vi "Process.vi"(8 "error in":errorcluster, 11 "Plugin in":refnum<class "Sequencer with Output Values.lvclass">) -> (0 "error out":errorcluster, 3 "Plugin out":refnum<class "Sequencer with Output Values.lvclass">)   [LabVIEW 2024, in "Sequencer with Output Values.lvlib" / "Sequencer with Output Values.lvclass"]
uses:
  Sequencer with Output Values.lvclass
  C:/Program Files/National Instruments/LabVIEW 2024/vi.lib/FlexLogger/SDK/PluginSDK.lvlibp/PEFClasses/SDK/Plugin/Plugin.lvclass
  Sequencer with Output Values.lvclass/Sequencer with Output Values.ctl
  <vilib>/FlexLogger/SDK/PluginSDK.lvlibp/PEFClasses/SDK/Plugin/DataHelpers/Write 1D DBL (NChan 1Sample).vi
  <vilib>/FlexLogger/SDK/PluginSDK.lvlibp/PEFClasses/SDK/Plugin/DataHelpers/Write 1D Bool (NChan 1 Sample).vi
  <vilib>/FlexLogger/SDK/PluginSDK.lvlibp/PEFClasses/SDK/Plugin/Plugin.lvclass
  C:/Program Files/National Instruments/LabVIEW 2024/vi.lib/FlexLogger/SDK/PluginSDK.lvlibp/PEFClasses/SDK/Processing Element/Processing Element.lvclass
  C:/dev/niflexlogger-plugins/plugins/Sequencer with Output Values/source/Sequencer with Output Values/Sequencer with Output Values.lvclass
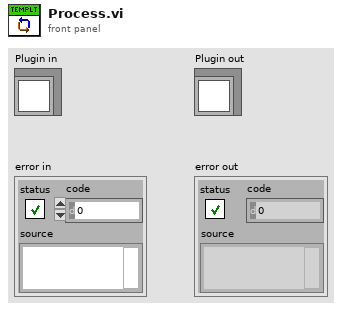
[diagram p1: front panel]
types:
  T1 = typedef "Sequencer with Output Values.lvlib/Sequencer with Output Values.lvclass/Params.ctl" = cluster{"Step Values":T2[], "Only Execute When Test Running":bool, "Current Sequence ID":u32, "Total Iterations":u32, "Last Timestamp":timestamp, "Number of Sequence Steps":i32, "Number of Analog Channels":i32, "Number of Digital Channels":i32, "Delay Before Starting Sequence":dbl}
  T2 = typedef "Step Settings.ctl" = cluster{"Duration":dbl, "Mode":string, "Delay Between Values":dbl, "Analog Values":string[], "Digital Values":string[]}
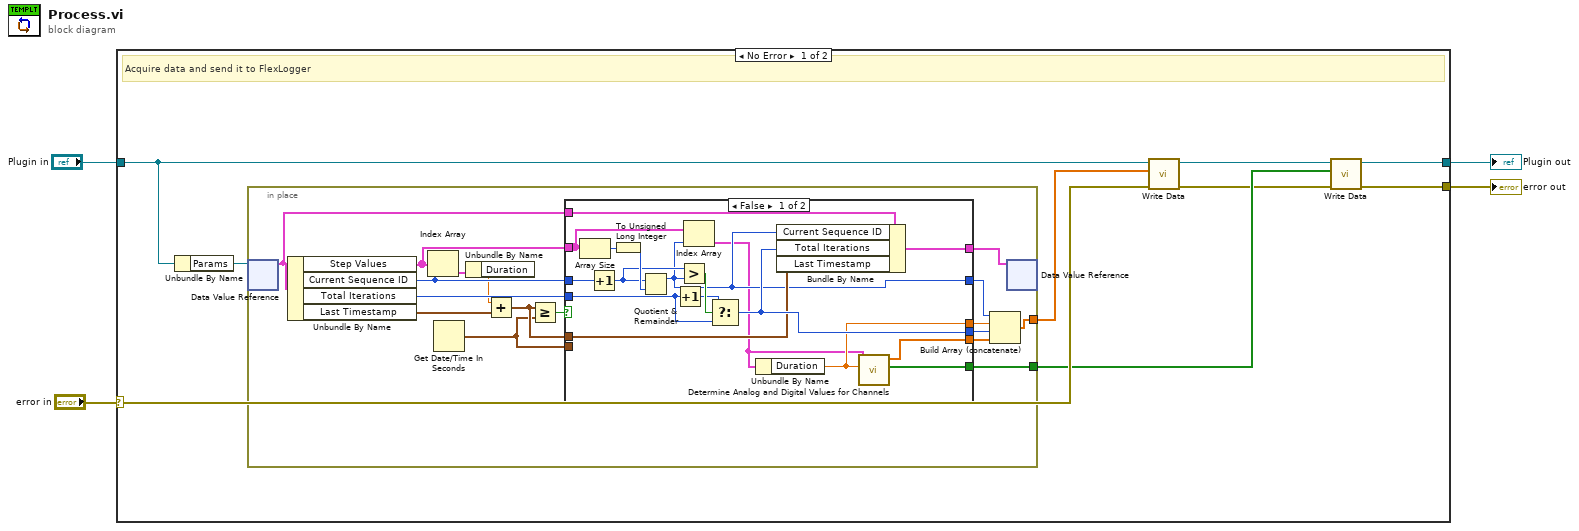
[diagram p0: block diagram]
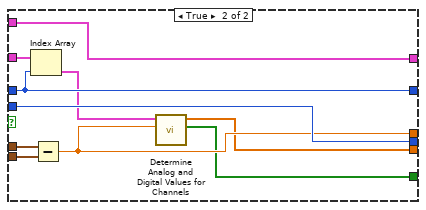
[diagram p2: hidden frame]
diagram:
  n1 = case shown="No Error" "error in" {
    selector: "error in" -> [w12 w58]
    tunnel: [w6 w59] -> w4
    tunnel: "Plugin in" -> [w13 w59]
    tunnel: [w5 w58] -> w1
    frame No Error {
      # "Acquire data and send it to FlexLogger"
      n2 = Unbundle By Name(w13) -> ("Params"=w11:refnum<data-value>)
      n3 = in-place {
        in-place-border: [w27] -> w10
        in-place-border: [w14] -> w8
        n4 = in-place-dvr #1(w11) -> (w30:T1)  [unwired: 1 out]
        n5 = Unbundle By Name(w30) -> ("Step Values"=w29:T2[], "Current Sequence ID"=w25:u32, "Total Iterations"=w28:u32, "Last Timestamp"=w23:timestamp)
        n6 = Index Array(array=w29, index=w25) -> (element=w21:T2)
        n7 = Get Date/Time In Seconds() -> (seconds since 1Jan1904=w17:timestamp)
        n8 = Unbundle By Name(w21) -> ("Duration"=w20:dbl)
        n9 = Add(x=w20, y=w23) -> (x+y=w18:timestamp)
        n10 = Greater Or Equal?(x=w18, y=w17) -> (x >= y?=w24:bool)
        n11 = case shown="False" w24 {
          tunnel: w30 -> [w42 w56]
          tunnel: w25 -> [w46 w52]
          tunnel: w29 -> [w36 w53]
          tunnel: w28 -> [w44 w57]
          tunnel: [w35 w52] -> w22
          tunnel: [w40 w57] -> w19
          tunnel: [w41 w56] -> w26
          tunnel: w18 -> [w37 w55]
          tunnel: w17 -> [_ w54]
          tunnel: [w32 w50] -> w16
          tunnel: [w34 w49] -> w15
          tunnel: [w33 w48] -> w14
          frame False {
            n12 = Array Size(array=w36) -> (size(s)=w47:i32)
            n13 = Increment(x=w46) -> (x+1=w38:u32)
            n14 = To Unsigned Long Integer(number=w47) -> (unsigned 32bit integer=w39:u32)
            n15 = Quotient & Remainder(x=w38, y=w39) -> (x-y*floor(x/y)=w35:u32)  [unwired: 1 out]
            n16 = Increment(x=w44) -> (x+1=w43:u32)
            n17 = Greater?(x=w38, y=w35) -> (0:w45:bool)
            n18 = Index Array(array=w36, index=w35) -> (element=w31:T2)
            n19 = Select(t=w43, s=w45, f=w44) -> (s? t:f=w40:u32)
            n20 = Unbundle By Name(w31) -> ("Duration"=w32:dbl)
            n21 = Bundle By Name(cluster=w42, "Current Sequence ID"=w35, "Total Iterations"=w40, "Last Timestamp"=w37) -> (w41:T1)
            n22 = call "Determine Analog and Digital Values for Channels.vi"("Remaining Time"=w32, "Step Settings"=w31) -> ("Digital Values to Write"=w33:bool[], "Analog Values to Write"=w34:dbl[])  [unwired: 8 in]
          }
          frame True {
            n23 = Index Array(array=w53, index=w52) -> (element=w51:T2)
            n24 = Subtract(x=w55, y=w54) -> (x-y=w50:dbl)
            n25 = call "Determine Analog and Digital Values for Channels.vi"("Remaining Time"=w50, "Step Settings"=w51) -> ("Digital Values to Write"=w48:bool[], "Analog Values to Write"=w49:dbl[])  [unwired: 8 in]
          }
        }
        n26 = Build Array (concatenate)(w22, w16, w19, w15) -> (w27:dbl[])
        n27 = in-place-dvr #1(w26) -> ()  [unwired: 2 out]
      }
      n28 = call-poly <vilib>:"Write Data.vi"("error in (no error)"=w12, "Data"=w10, "Plugin in"=w13) -> ("error out"=w7:errorcluster, "Plugin out"=w9:refnum<class "Sequencer with Output Values.lvclass">)  [unwired: 7 in]
      n29 = call-poly <vilib>:"Write Data.vi"("error in (no error)"=w7, "Data"=w8, "Plugin in"=w9) -> ("error out"=w5:errorcluster, "Plugin out"=w6:refnum<class "Sequencer with Output Values.lvclass">)  [unwired: 7 in]
    }
    frame Error {
    }
  }
  "error out" <- w1
  "Plugin out" <- w4
